vi "Joints FGV.vi"(6 "Command":enum16{"Get", "Initialize", "Set"}(ring), 8 "error in (no error)":errorcluster, 10 "Joint Points":variant) -> (0 "error out":errorcluster, 2 "Joint Points":variant)   [LabVIEW 2014]
panel:
  out "Bodies":variant[](array[variant])
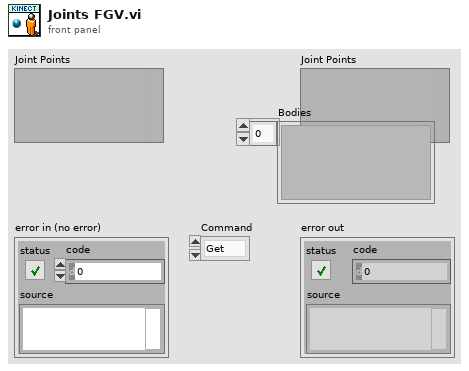
[diagram p1: front panel]
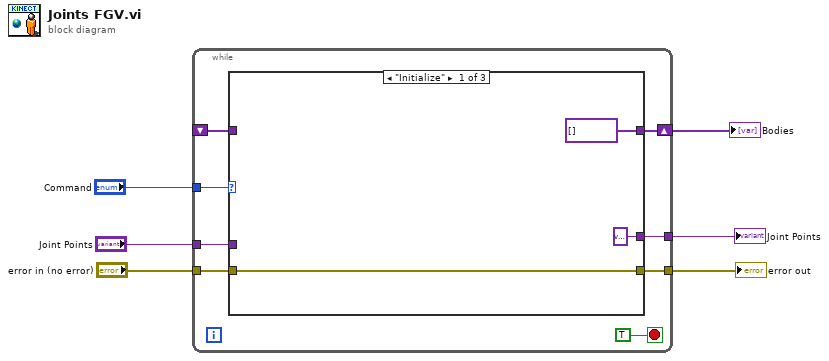
[diagram p0: block diagram]
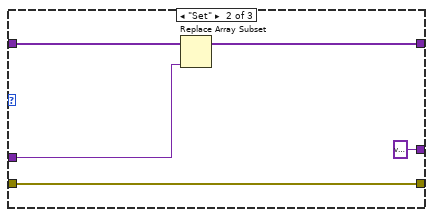
[diagram p2: hidden frame]
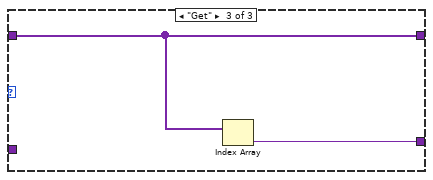
[diagram p3: hidden frame]
diagram:
  n1 = while {
    tunnel: "Command" -> [w13]
    shift-right: [w12] -> w1
    shift-left: _ -> [w11]
    tunnel: "error in (no error)" -> [w10]
    tunnel: [w9] -> w4
    tunnel: [w8] -> w2
    tunnel: "Joint Points" -> [w7]
    stop <- TRUE stop-if-true
    n2 = case shown="\"Initialize\"" w13 {
      tunnel: [variant[] [] w19 w24] -> w12
      tunnel: w11 -> [_ w21 w24]
      tunnel: w10 -> [w16 w18 _]
      tunnel: [w16 w18 _] -> w9
      tunnel: [variant ("Joint Points") variant w23] -> w8
      tunnel: w7 -> [_ w20 _]
      frame "Initialize" {
      }
      frame "Set" {
        n3 = Replace Array Subset(array=w21, new element=w20) -> (w19:variant[])  [unwired: 1 in]
      }
      frame "Get" {
        n4 = Index Array(array=w24) -> (element=w23:variant)  [unwired: 1 in]
      }
    }
  }
  "error out" <- w4
  "Joint Points" <- w2
  "Bodies" <- w1
